vi "WT300 Calculate Crest Factor.vi"(11 "All Data":dbl[](array[numeric])) -> (2 "Voltage Crest Factor":dbl, 3 "Current Crest Factor":dbl)   [LabVIEW 2016]
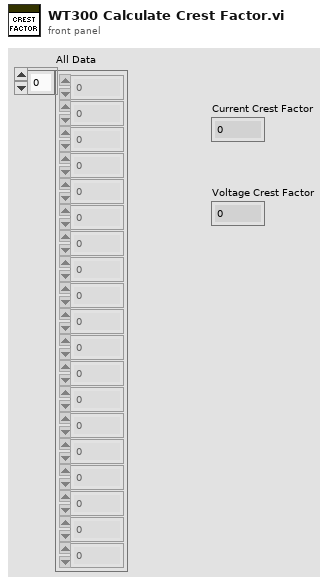
[diagram p1: front panel]
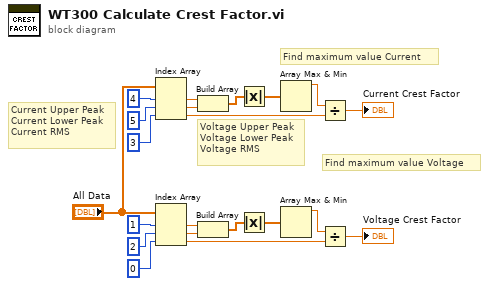
[diagram p0: block diagram]
diagram:
  # "Find maximum value Current"
  # "Find maximum value Voltage"
  # "Current Upper Peak\nCurrent Lower Peak\nCurrent RMS"
  # "Voltage Upper Peak\nVoltage Lower Peak\nVoltage RMS"
  n1 = Index Array(array="All Data", index #1=4 ("index"), index #2=5 ("index"), index #3=3 ("index")) -> (element #1=w18:dbl, element #2=w5:dbl, element #3=w3:dbl)
  n2 = Index Array(array="All Data", index #1=1 ("index"), index #2=2 ("index"), index #3=0 ("index")) -> (element #1=w21:dbl, element #2=w7:dbl, element #3=w1:dbl)
  n3 = Build Array(w18, w5) -> (w17:dbl[])
  n4 = Build Array(w21, w7) -> (w20:dbl[])
  n5 = Absolute Value(x=w17) -> (abs(x)=w16:dbl[])
  n6 = Absolute Value(x=w20) -> (abs(x)=w19:dbl[])
  n7 = Array Max & Min(array=w16) -> (max value=w13:dbl)  [unwired: 3 out]
  n8 = Array Max & Min(array=w19) -> (max value=w11:dbl)  [unwired: 3 out]
  n9 = Divide(x=w13, y=w3) -> (x/y=→"Current Crest Factor":dbl)
  n10 = Divide(x=w11, y=w1) -> (x/y=→"Voltage Crest Factor":dbl)
